vi "IOControls.Compile.vi"(8 "error in (no error)":errorcluster, 11 "Section Ref in":T4 format="%.0x") -> (0 "error out":errorcluster, 2 "Settings":T1 {"Signal.Cmd.Refs"."Signal Refs" format="%.0x"; "Signal.Cmd.Info"."Signals"."Byte Order" items=["Little Endian", "Big Endian"]; "Signal.Cmd.Info"."Signals"."Data Type" items=["Signed", "Unsigned", "IEEE Float"]; "Settings.Refs"."Signal Refs" format="%.0x"; "Signal.Resp.Refs"."Signal Refs" format="%.0x"; "Signal.Resp.Info"."Signals"."Byte Order" items=["Little Endian", "Big Endian"]; "Signal.Resp.Info"."Signals"."Data Type" items=["Signed", "Unsigned", "IEEE Float"]; "Trigger.Refs"."Signal Refs" format="%.0x"; "Status.Refs"."Signal Refs" format="%.0x"}, 3 "Section Ref out":T4 format="%.0x")   [LabVIEW 2024, in "Diagnostics Addon System Explorer.lvlib"]
uses:
  Diagnostics Addon System Explorer.lvlib
  <vilib>/NI VeriStand/Custom Device API/Custom Device Item Ref.ctl
  Types/Service.Export.ctl
  Types/Frame.Ref.ctl
  Addon Shared/Types/Type.ctl
  Addon Shared/Types/Frame.Compile.ctl
  Addon Shared/Types/Signal.ctl
  Types/FG.Action.ctl
  Signal.FG.vi
  Frame.GetSignalRefs.vi
  Addon Shared/SubVIs/Constants.vi
  <vilib>/NI VeriStand/Custom Device Tools/Custom Device Utility Library/NI VeriStand - Search for Item by GUID.vi
  <vilib>/NI VeriStand/Custom Device Tools/Custom Device Utility Library/NI VeriStand - Search for Item by Name.vi
  <vilib>/NI/NI VeriStand Advanced SysDef API/SysDef API/SysDef.Property.Set.vi
  <vilib>/NI/NI VeriStand Advanced SysDef API/_SubVIs/SysDef.Property.Set.U32.vi
  <vilib>/NI VeriStand/Custom Device API/NI VeriStand - Get Item Property.vi
  <vilib>/NI VeriStand/Custom Device API/Get Item Property (U32).vi
  <vilib>/NI VeriStand/Custom Device API/NI VeriStand - Get Item Data.vi
  <vilib>/NI/NI VeriStand Advanced SysDef API/_SubVIs/SysDef.Property.Set.DBL.vi
  <vilib>/NI/NI VeriStand Advanced SysDef API/_SubVIs/SysDef.Property.Set.String.vi
  <vilib>/NI VeriStand/Custom Device API/Get Item Property (Double).vi
  <vilib>/NI VeriStand/Custom Device API/Get Item Property (String).vi
  <vilib>/NI VeriStand/Custom Device API/NI VeriStand - Get Custom Device Channel Data.vi
  <vilib>/NI VeriStand/Custom Device Tools/Custom Device Utility Library/Custom Device Utility Library.lvlib
  <vilib>/NI VeriStand/Custom Device API/Custom Device API.lvlib
  Addon Shared/Diagnostics Addon Shared.lvlib
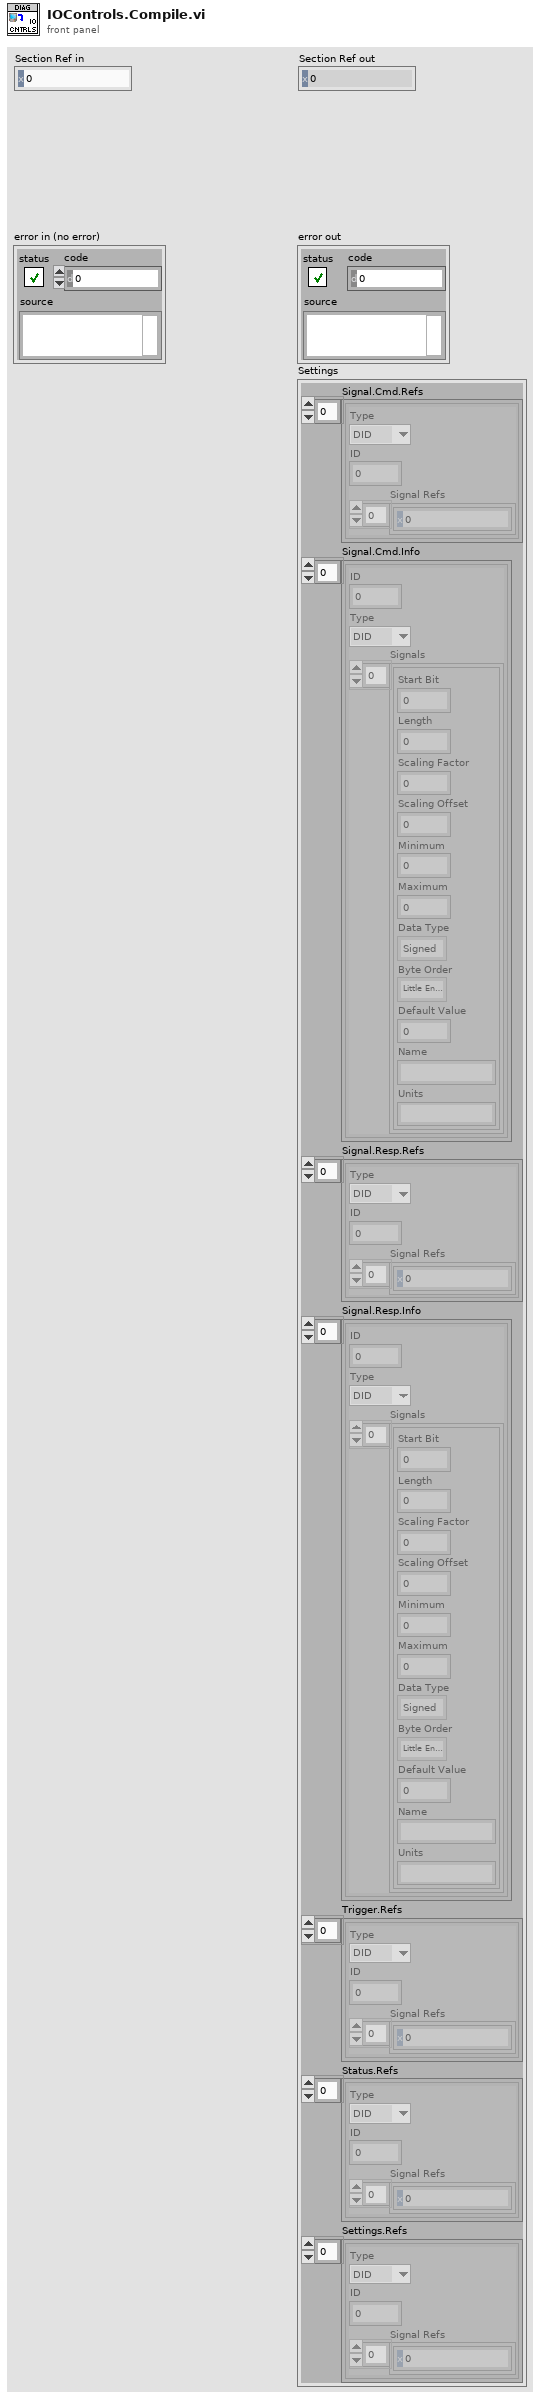
[diagram p1: front panel]
types:
  T1 = typedef "Diagnostics Addon System Explorer.lvlib/Service.Export.ctl" = cluster{"Signal.Cmd.Refs":T2[], "Signal.Cmd.Info":T5[], "Signal.Resp.Refs":T2[], "Signal.Resp.Info":T5[], "Trigger.Refs":T2[], "Status.Refs":T2[], "Settings.Refs":T2[]}
  T2 = typedef "Diagnostics Addon System Explorer.lvlib/Frame.Ref.ctl" = cluster{"Type":T3, "ID":u32, "Signal Refs":T4[]}
  T3 = typedef "Diagnostics Addon Shared.lvlib/Type.ctl" = enum16{"DID", "CDID", "PID", "CPID", "Read Memory", "Write Memory", "IO Control", "Routine Start", "Routine Request", "Routine Stop", "User Defined", "DTC Control", "Clear DTCs", "Read DTCs", "Start DTCs", "DTC Change Count", "Tester Present", "Unlock ECU", "Reset ECU", "Diag Session Control", "Communication Control", "DPID Control", "Poll Control", "Diag Comm Port Control"}
  T4 = typedef "Custom Device API.lvlib/Custom Device Item Ref.ctl" = u64
  T5 = typedef "Diagnostics Addon Shared.lvlib/Frame.Compile.ctl" = cluster{"ID":u32, "Type":T3, "Signals":T6[]}
  T6 = typedef "Diagnostics Addon Shared.lvlib/Signal.ctl" = cluster{"Start Bit":u32, "Length":u32, "Scaling Factor":dbl, "Scaling Offset":dbl, "Minimum":dbl, "Maximum":dbl, "Data Type":u32, "Byte Order":u32, "Default Value":dbl, "Name":string, "Units":string}
  T7 = typedef "Diagnostics Addon System Explorer.lvlib/FG.Action.ctl" = enum16{"Get", "Set"}
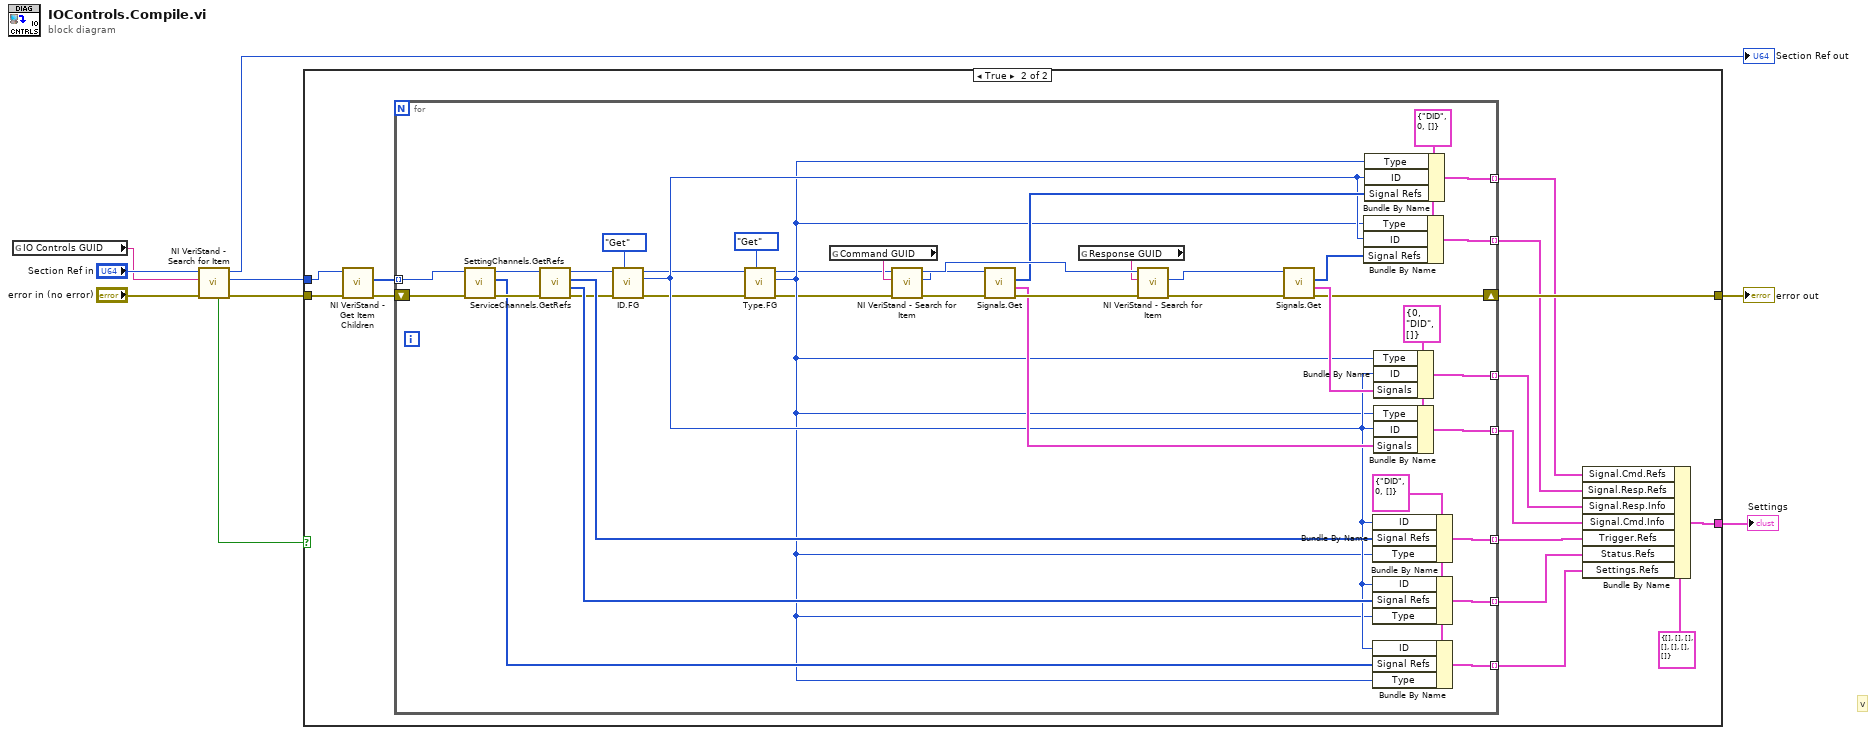
[diagram p0: block diagram]
diagram:
  # "v"
  n1 = global read "Constants.vi" "IO Controls GUID"() -> (w2:string)
  n2 = call-poly <vilib>:"NI VeriStand - Search for Item.vi"("error in"="error in (no error)", "Item GUID"=w2, "Section Ref in"="Section Ref in") -> ("error out"=w4:errorcluster, "Item Ref"=w5:T4, "Section Ref out"=→"Section Ref out":T4, "Found"=w3:bool)  [unwired: 5 in]
  n3 = case shown="True" w3 {
    tunnel: [w10 w24] -> w8
    tunnel: w5 -> [_ w21]
    tunnel: w4 -> [w10 w20]
    tunnel: [_ w12] -> w1
    frame False {
    }
    frame True {
      n4 = call <vilib>:"NI VeriStand - Get Item Children.vi"("error in (no error)"=w20, "Item Ref in"=w21) -> ("error out"=w22:errorcluster, "Child Refs"=w23:T4[])  [unwired: 6 in, 2 out]
      n5 = for {
        shift-right: [w56] -> w24
        shift-left: w22 -> [w41]
        tunnel: w23 -> [w42] mode=indexing
        tunnel: [w55] -> w16 mode=indexing
        tunnel: [w54] -> w15 mode=indexing
        tunnel: [w50] -> w18 mode=indexing
        tunnel: [w49] -> w17 mode=indexing
        tunnel: [w43] -> w14 mode=indexing
        tunnel: [w38] -> w13 mode=indexing
        tunnel: [w36] -> w11 mode=indexing
        w37 = T2 {"Type"=enum."DID", "ID"=0, "Signal Refs"=[]} ("cluster")
        w52 = T2 {"Type"=enum."DID", "ID"=0, "Signal Refs"=[]} ("Cmd")
        w64 = T5 {"ID"=0, "Type"=enum."DID", "Signals"=[]} ("PID In")
        n6 = call "SettingChannels.GetRefs.vi"("error in (no error)"=w41, "Item Ref in"=w42) -> ("error out"=w40:errorcluster, "Settings"=w34:T4[], "Section Ref out"=w39:T4)  [unwired: 7 in]
        n7 = call "ServiceChannels.GetRefs.vi"("error in (no error)"=w40, "Item Ref in"=w39) -> ("error out"=w44:errorcluster, "Status"=w47:T4[], "Trigger"=w46:T4[], "Section Ref out"=w45:T4)  [unwired: 6 in]
        n8 = call "ID.FG.vi"("Action"=FG.Action."Get", "error in (no error)"=w44, "Device Item Ref in"=w45) -> ("error out"=w28:errorcluster, "ID"=w35:u32, "Device Item Ref out"=w27:T4)  [unwired: 6 in]
        n9 = call "Type.FG.vi"("Action"=FG.Action."Get", "error in (no error)"=w28, "Device Item Ref in"=w27) -> ("error out"=w25:errorcluster, "Type"=w29:T3, "Device Item Ref out"=w26:T4)  [unwired: 6 in]
        n10 = global read "Constants.vi" "Command GUID"() -> (w59:string)
        n11 = call-poly <vilib>:"NI VeriStand - Search for Item.vi"("error in"=w25, "Item GUID"=w59, "Section Ref in"=w26) -> ("error out"=w30:errorcluster, "Item Ref"=w31:T4, "Section Ref out"=w62:T4)  [unwired: 5 in, 1 out]
        n12 = call "Signals.Get.vi"("error in (no error)"=w30, "Device Item Ref out"=w31) -> ("error out"=w63:errorcluster, "Parameters"=w58:T6[], "Child Refs"=w53:T4[])  [unwired: 6 in, 1 out]
        n13 = global read "Constants.vi" "Response GUID"() -> (w61:string)
        n14 = call-poly <vilib>:"NI VeriStand - Search for Item.vi"("error in"=w63, "Item GUID"=w61, "Section Ref in"=w62) -> ("error out"=w32:errorcluster, "Item Ref"=w33:T4)  [unwired: 5 in, 2 out]
        n15 = call "Signals.Get.vi"("error in (no error)"=w32, "Device Item Ref out"=w33) -> ("error out"=w56:errorcluster, "Parameters"=w57:T6[], "Child Refs"=w51:T4[])  [unwired: 6 in, 1 out]
        n16 = Bundle By Name(cluster=w52, "Type"=w29, "ID"=w35, "Signal Refs"=w51) -> (w49:T2)
        n17 = Bundle By Name(cluster=w52, "Type"=w29, "ID"=w35, "Signal Refs"=w53) -> (w50:T2)
        n18 = Bundle By Name(cluster=w37, "ID"=w35, "Signal Refs"=w46, "Type"=w29) -> (w43:T2)
        n19 = Bundle By Name(cluster=w37, "ID"=w35, "Signal Refs"=w47, "Type"=w29) -> (w38:T2)
        n20 = Bundle By Name(cluster=w37, "ID"=w35, "Signal Refs"=w34, "Type"=w29) -> (w36:T2)
        n21 = Bundle By Name(cluster=w64, "Type"=w29, "ID"=w35, "Signals"=w57) -> (w55:T5)
        n22 = Bundle By Name(cluster=w64, "Type"=w29, "ID"=w35, "Signals"=w58) -> (w54:T5)
      }
      n23 = Bundle By Name(cluster=T1 {"Signal.Cmd.Refs"=[], "Signal.Cmd.Info"=[], "Signal.Resp.Refs"=[], "Signal.Resp.Info"=[], "Trigger.Refs"=[], "Status.Refs"=[], "Settings.Refs"=[]} ("Settings"), "Signal.Cmd.Refs"=w18, "Signal.Resp.Refs"=w17, "Signal.Resp.Info"=w16, "Signal.Cmd.Info"=w15, "Trigger.Refs"=w14, "Status.Refs"=w13, "Settings.Refs"=w11) -> (w12:T1)
    }
  }
  "error out" <- w8
  "Settings" <- w1
